vi "Update Scalar Channels.vi"(8 "error in (no error)":errorcluster, 11 "valid scalar channels":T1[](array[typedef]) {"Item Ref" format="%.0x"}) -> (0 "error out":errorcluster)   [LabVIEW 2018, in "FPGA Addon System Explorer.lvlib"]
uses:
  FPGA Addon System Explorer.lvlib
  Types/Output Scalar.ctl
  Addon Shared/Types/FPGA Addon Data Type.ctl
  <vilib>/NI Veristand/Custom Device API/Custom Device Item Ref.ctl
  Addon Shared/Types/Register Information.ctl
  Addon Shared/Types/FG Action.ctl
  Addon Shared/SubVIs/Constants.vi
  <vilib>/NI/NI VeriStand Advanced SysDef API/SysDef API/SysDef.Property.Get.vi
  <vilib>/NI/NI VeriStand Advanced SysDef API/_SubVIs/SysDef.Property.Get.Variant.vi
  <vilib>/NI/NI VeriStand Advanced SysDef API/SysDef API/SysDef.Property.Set.vi
  <vilib>/NI/NI VeriStand Advanced SysDef API/_SubVIs/SysDef.Property.Set.Variant.vi
  <vilib>/NI Veristand/Custom Device API/Custom Device API.lvlib
  Addon Shared/FPGA Addon Shared.lvlib
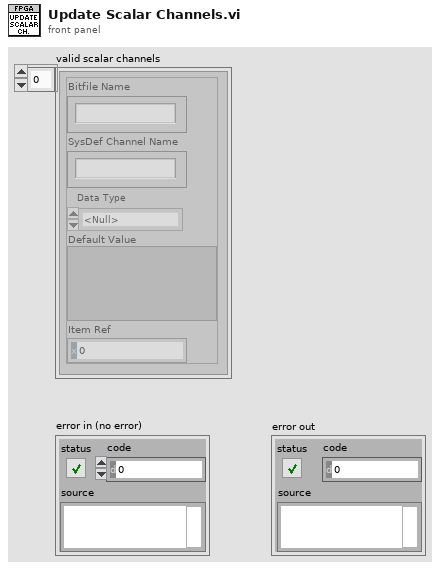
[diagram p1: front panel]
types:
  T1 = typedef "FPGA Addon System Explorer.lvlib/Output Scalar.ctl" = cluster{"Bitfile Name":string, "SysDef Channel Name":string, "Data Type":T2, "Default Value":variant, "Item Ref":T3}
  T2 = typedef "FPGA Addon Shared.lvlib/FPGA Addon Data Type.ctl" = enum8{"<Null>", "I8", "I16", "I32", "I64", "U8", "U16", "U32", "U64", "SGL", "Boolean", "Analog PWM In Settings", "Analog PWM In", "Digital PWM In Settings", "Digital PWM In", "Digital PWM Out", "Sine Out", "FXP", "FXP+/-24.5", "FXP+/-16.5", "FXP+/-32.8", "FXP+/-64.32", "FXP+/-16.7", "FXP+/-20.5", "FXP+/-27.5", "FXP+/-32.16", "FXP+16.3", "FXP+18.3", "Digital Static In", "Digital Static Out", "Digital Static In Settings", "Digital WSS Out", "Quad Encoder Settings", "Quad Encoder In", "Group"}
  T3 = typedef "Custom Device API.lvlib/Custom Device Item Ref.ctl" = u64
  T4 = typedef "FPGA Addon Shared.lvlib/Register Information.ctl" = cluster{"Name":string, "Data Type":T2, "Default Value":variant, "Attributes":variant}
  T5 = typedef "FPGA Addon Shared.lvlib/FG Action.ctl" = enum8{"GET", "SET"}
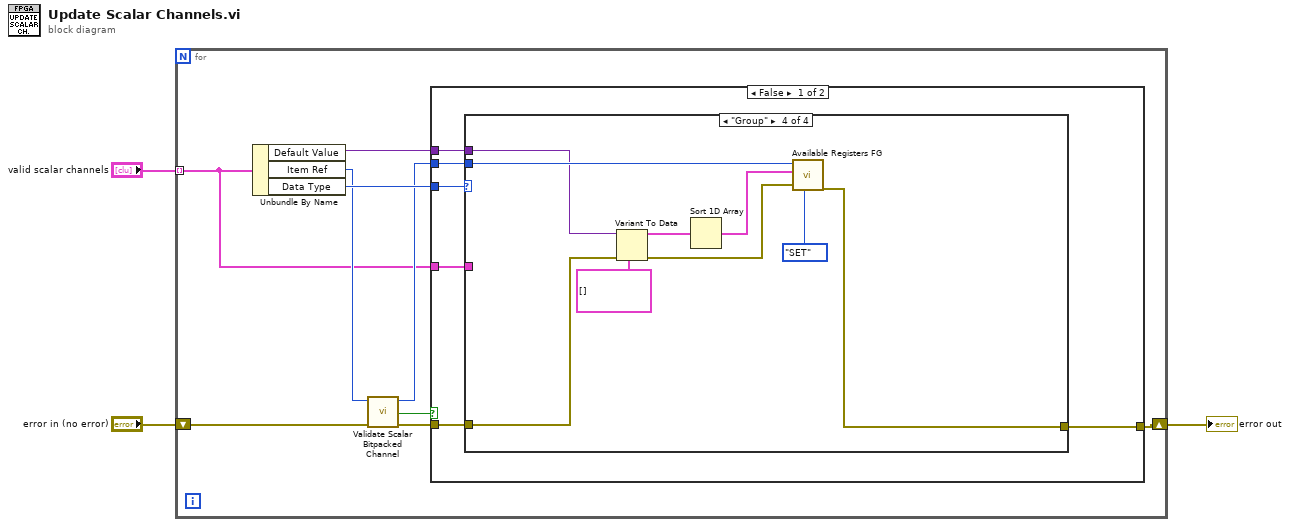
[diagram p0: block diagram]
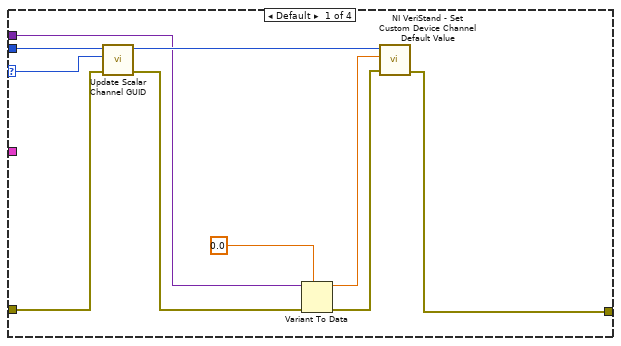
[diagram p2: hidden frame]
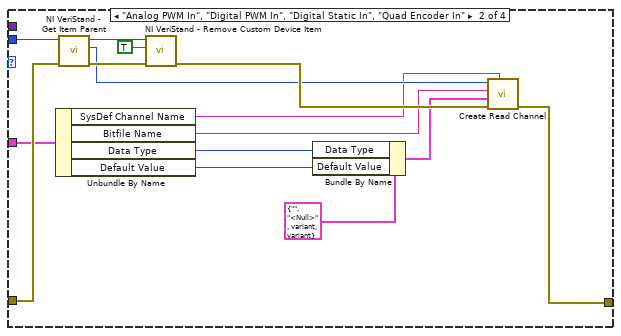
[diagram p3: hidden frame]
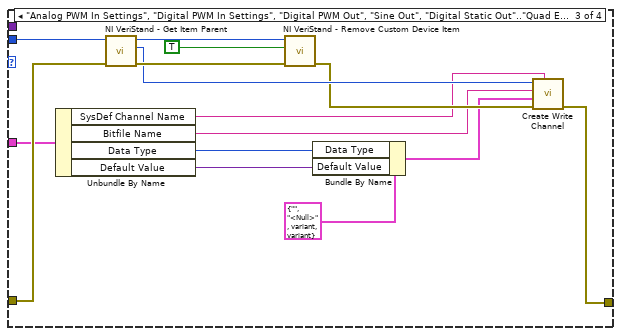
[diagram p4: hidden frame]
diagram:
  n1 = for {
    shift-right: [w12] -> w2
    shift-left: "error in (no error)" -> [w9]
    tunnel: "valid scalar channels" -> [w4] mode=indexing
    n2 = Unbundle By Name(w4) -> ("Default Value"=w10:variant, "Item Ref"=w8:T3, "Data Type"=w11:T2)
    n3 = call "Validate Scalar Bitpacked Channel.vi"("error in (no error)"=w9, "Item Ref"=w8) -> ("error out"=w6:errorcluster, "bitpacked"=w5:bool, "item ref out"=w7:T3)  [unwired: 7 in]
    n4 = case shown="False" w5 {
      tunnel: [w18 w68] -> w12
      tunnel: w11 -> [w16 _]
      tunnel: w10 -> [w15 _]
      tunnel: w7 -> [w14 _]
      tunnel: w6 -> [w17 w68]
      tunnel: w4 -> [w13 _]
      frame False {
        n5 = case shown="\"Group\"" w16 {
          selector: w16 -> [w22 _ _ _]
          tunnel: w14 -> [w24 w43 w58 w66]
          tunnel: w17 -> [w23 w42 w57 w62]
          tunnel: [w25 w34 w46 w64] -> w18
          tunnel: w15 -> [w19 _ _ w63]
          tunnel: w13 -> [_ w37 w50 _]
          frame Default {
            n6 = call "Update Scalar Channel GUID.vi"("error in (no error)"=w23, "Data Type"=w22, "item ref in"=w24) -> ("error out"=w21:errorcluster, "item ref out"=w20:T3)  [unwired: 7 in]
            n7 = Variant To Data(error in=w21, type=0.0, Variant=w19) -> (data=w27:dbl, error out=w26:errorcluster)
            n8 = call <vilib>:"NI VeriStand - Set Custom Device Channel Default Value.vi"("error in (no error)"=w26, "Default Value"=w27, "Channel Ref in"=w20) -> ("error out"=w25:errorcluster)  [unwired: 7 in, 1 out]
          }
          frame "Analog PWM In", "Digital PWM In", "Digital Static In", "Quad Encoder In" {
            n9 = Unbundle By Name(w37) -> ("SysDef Channel Name"=w29:string, "Bitfile Name"=w31:string, "Data Type"=w36:T2, "Default Value"=w35:variant)
            n10 = call <vilib>:"NI VeriStand - Get Item Parent.vi"("error in (no error)"=w42, "Item Ref in"=w43) -> ("error out"=w39:errorcluster, "Parent Ref"=w30:T3, "Item Ref out"=w41:T3)  [unwired: 6 in, 1 out]
            n11 = call <vilib>:"NI VeriStand - Remove Custom Device Item.vi"("error in (no error)"=w39, "Force Delete (F)"=TRUE, "Item Ref in"=w41) -> ("error out"=w33:errorcluster)  [unwired: 7 in, 1 out]
            n12 = Bundle By Name(cluster=T4 {"Name"="", "Data Type"=enum."<Null>", "Default Value"=variant, "Attributes"=variant} ("Cluster"), "Data Type"=w36, "Default Value"=w35) -> (w32:T4)
            n13 = call "Create Read Channel.vi"("Name"=w29, "error in (no error)"=w33, "Channel"=w32, "Bitfile Name"=w31, "Item Ref in"=w30) -> ("error out"=w34:errorcluster)  [unwired: 6 in]
          }
          frame "Analog PWM In Settings", "Digital PWM In Settings", "Digital PWM Out", "Sine Out", "Digital Static Out".."Quad Encoder Settings" {
            n14 = Unbundle By Name(w50) -> ("SysDef Channel Name"=w44:string, "Bitfile Name"=w45:string, "Data Type"=w49:T2, "Default Value"=w48:variant)
            n15 = call <vilib>:"NI VeriStand - Get Item Parent.vi"("error in (no error)"=w57, "Item Ref in"=w58) -> ("error out"=w54:errorcluster, "Parent Ref"=w53:T3, "Item Ref out"=w56:T3)  [unwired: 6 in, 1 out]
            n16 = call <vilib>:"NI VeriStand - Remove Custom Device Item.vi"("error in (no error)"=w54, "Force Delete (F)"=TRUE, "Item Ref in"=w56) -> ("error out"=w52:errorcluster)  [unwired: 7 in, 1 out]
            n17 = Bundle By Name(cluster=T4 {"Name"="", "Data Type"=enum."<Null>", "Default Value"=variant, "Attributes"=variant} ("Cluster"), "Data Type"=w49, "Default Value"=w48) -> (w47:T4)
            n18 = call "Create Write Channel.vi"("Name"=w44, "error in (no error)"=w52, "Cluster"=w47, "Bitfile Name"=w45, "Item Ref in"=w53) -> ("error out"=w46:errorcluster)  [unwired: 6 in]
          }
          frame "Group" {
            n19 = Variant To Data(error in=w62, type=T4[] [], Variant=w63) -> (data=w60:T4[], error out=w61:errorcluster)
            n20 = Sort 1D Array(array=w60) -> (sorted array=w59:T4[])
            n21 = call "Available Registers FG.vi"("Action"=FG_Action."SET", "error in (no error)"=w61, "Available Registers"=w59, "Item Ref"=w66) -> ("error out"=w64:errorcluster)  [unwired: 5 in, 2 out]
          }
        }
      }
      frame True {
      }
    }
  }
  "error out" <- w2
